vi "roundToNearestX.vi"(0 "Numeric":dbl, 1 "Round to Nearest":dbl, 2 "Array":dbl[](array[numeric])) -> (3 "roundNearest":dbl, 4 "roundedArray":dbl[](array[numeric]))   [LabVIEW 2022 SP3]
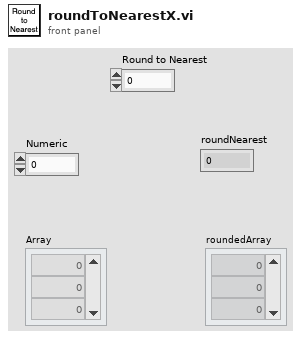
[diagram p1: front panel]
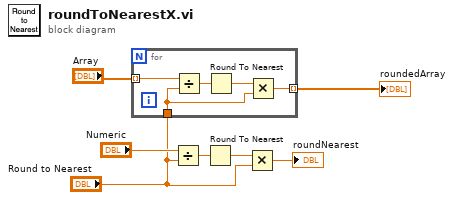
[diagram p0: block diagram]
diagram:
  n1 = for {
    tunnel: "Round to Nearest" -> [w8]
    tunnel: "Array" -> [w10] mode=indexing
    tunnel: [w9] -> w1 mode=indexing
    n2 = Divide(x=w10, y=w8) -> (x/y=w12:dbl)
    n3 = Round To Nearest(number=w12) -> (nearest integer value=w11:dbl)
    n4 = Multiply(x=w11, y=w8) -> (x*y=w9:dbl)
  }
  "roundedArray" <- w1
  n5 = Divide(x="Numeric", y="Round to Nearest") -> (x/y=w4:dbl)
  n6 = Round To Nearest(number=w4) -> (nearest integer value=w6:dbl)
  n7 = Multiply(x=w6, y="Round to Nearest") -> (x*y=→"roundNearest":dbl)
